vi "VI Tree.vi"   [LabVIEW 2020, in "Keysight DAQ970.lvlib"]
doc: "The VI Tree displays all the user-callable VIs of the instrument driver in an organized table."
uses:
  Keysight DAQ970.lvlib
panel:
  # "DAQ970"
  # "1.0.1"
  # "SEE DIAGRAM\nFOR VI Tree"
  # "© Keysight Technologies 2020 - 2021"
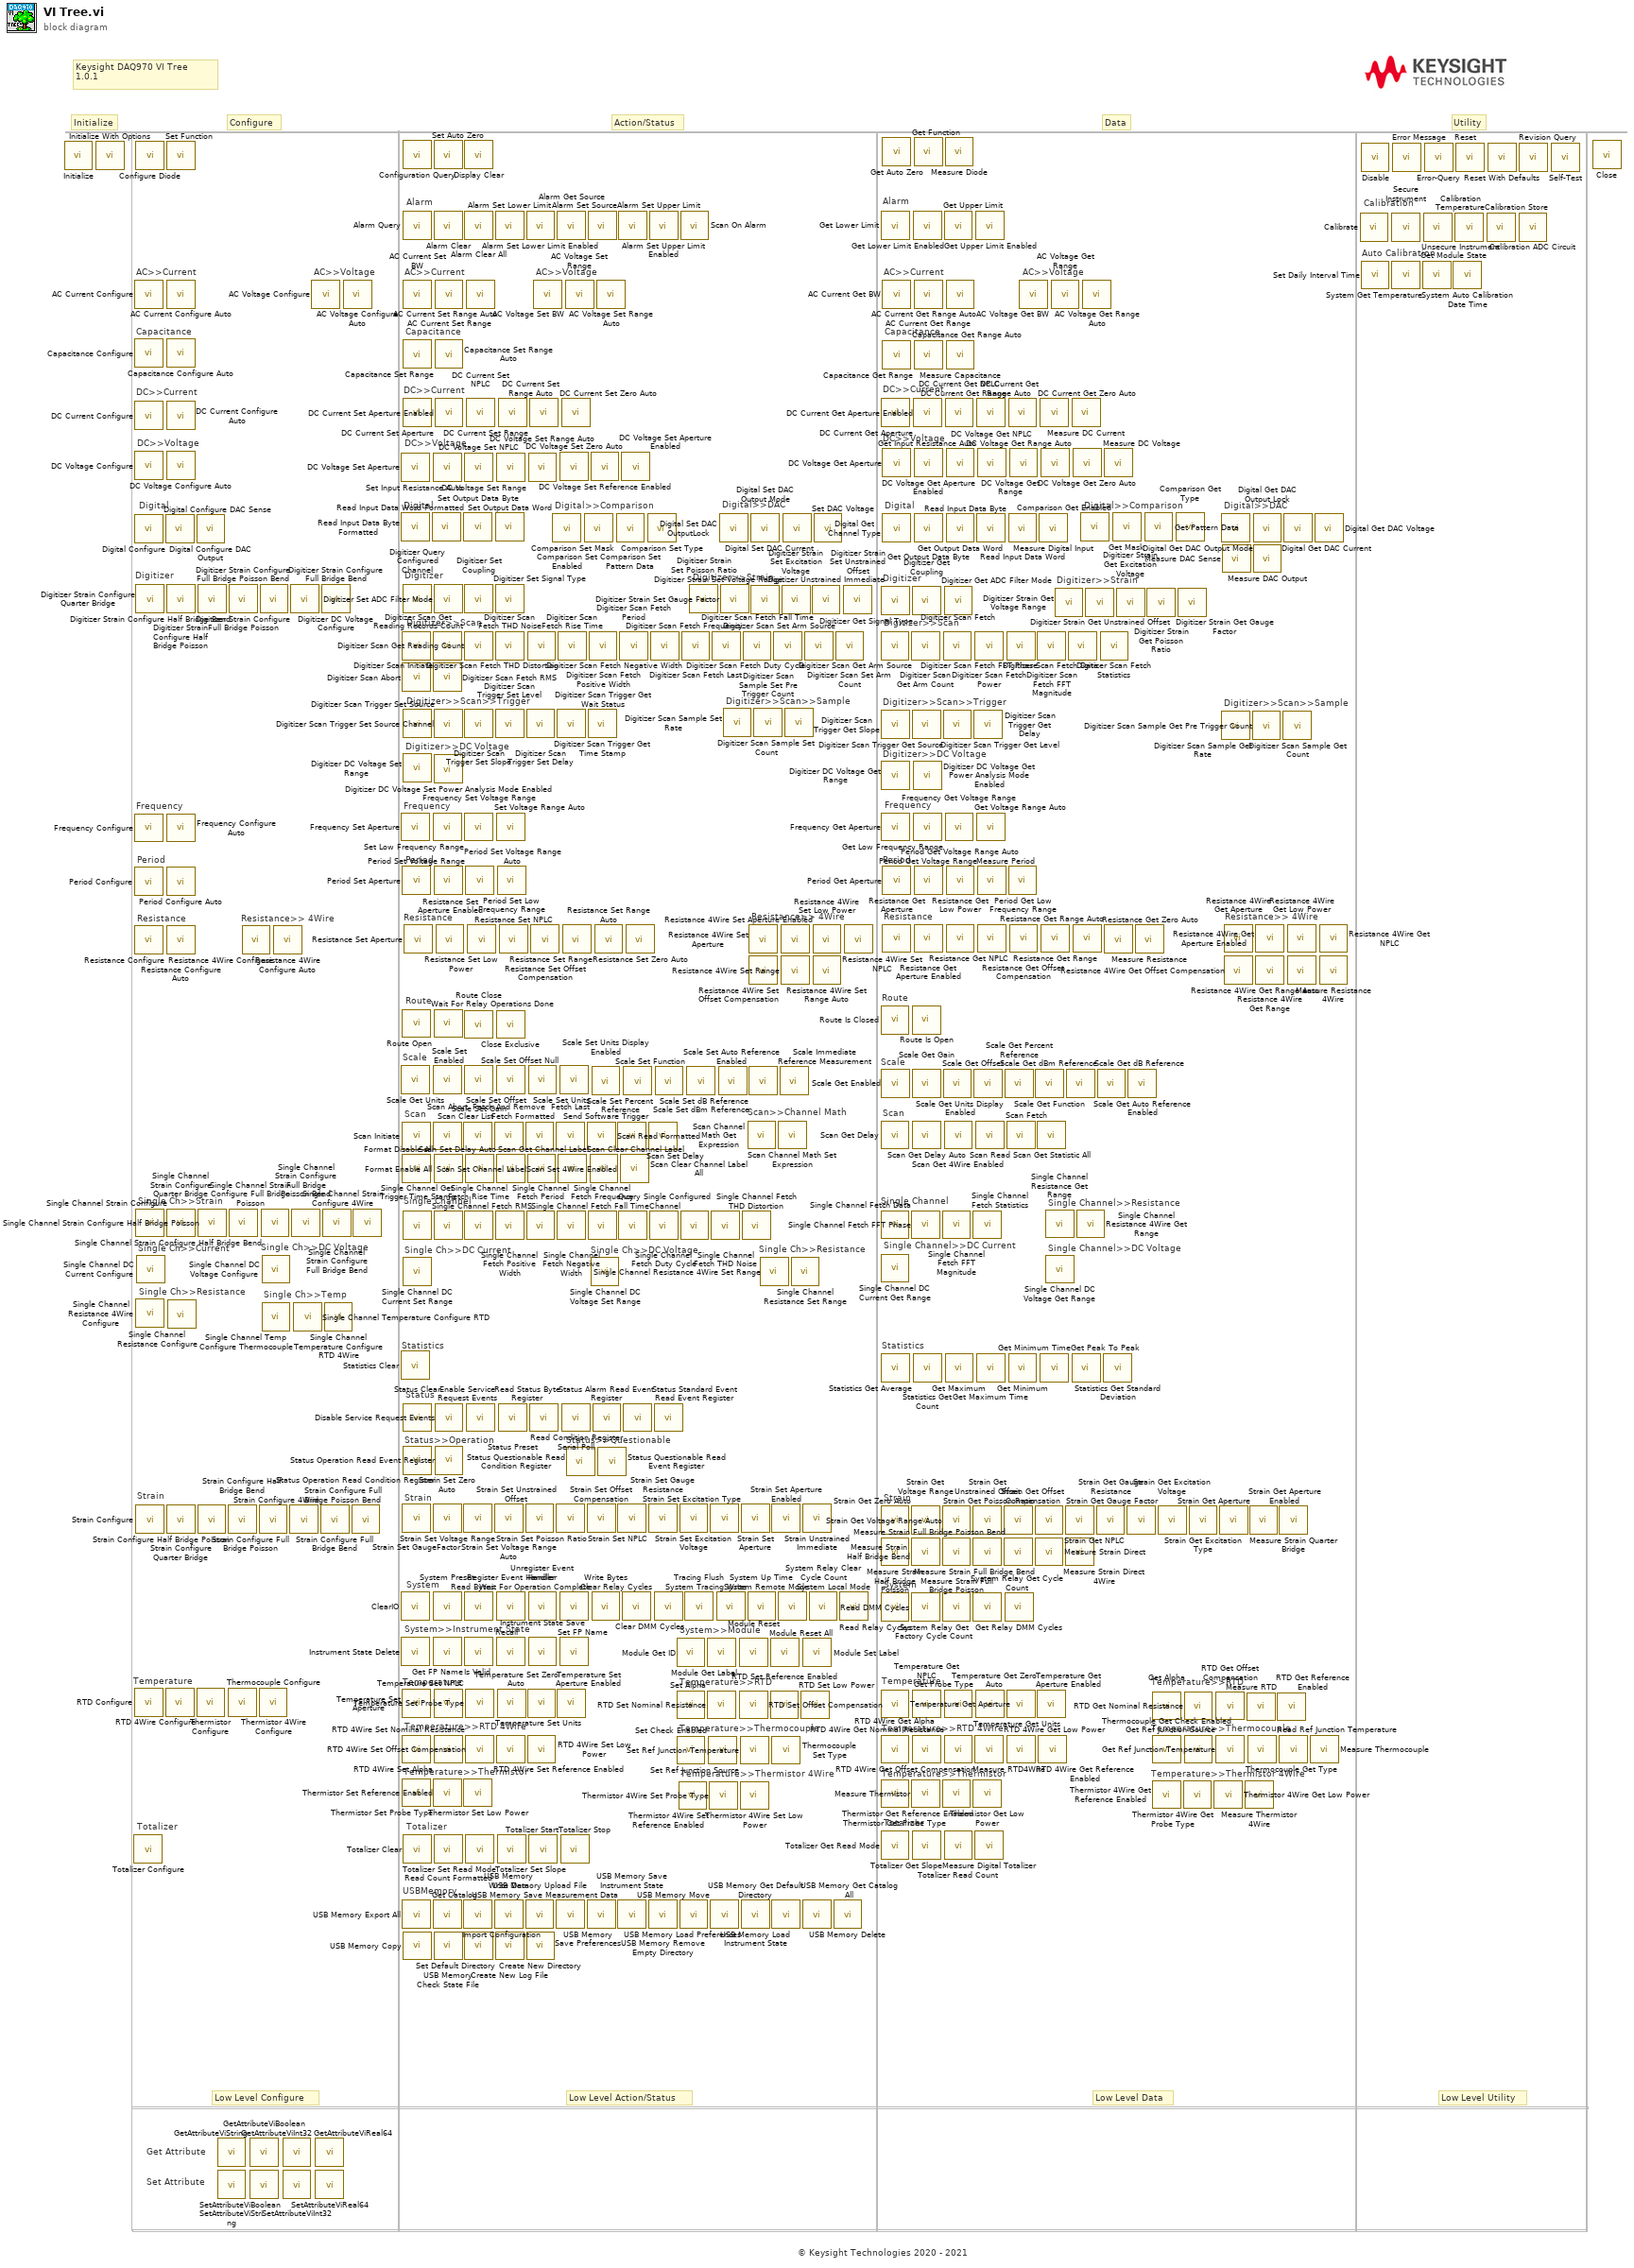
[diagram p0: block diagram]
diagram:
  # "Statistics"
  # "USBMemory"
  # "Totalizer"
  # "Totalizer"
  # "Temperature>>Thermistor"
  # "Temperature>>Thermistor 4Wire"
  # "Temperature>>Thermocouple"
  # "Temperature>>Thermistor 4Wire"
  # "Temperature>>Thermistor"
  # "Temperature>>Thermocouple"
  # "Temperature>>RTD 4Wire"
  # "Temperature>>RTD 4Wire"
  # "Temperature>>RTD"
  # "Temperature>>RTD"
  # "Temperature"
  # "Temperature"
  # "System>>Module"
  # "System>>Instrument State"
  # "Auto Calibration"
  # "System"
  # "System"
  # "Strain"
  # "Strain"
  # "Strain"
  # "Status>>Questionable"
  # "Status"
  # "Single Ch>>Temp"
  # "Single Ch>>Resistance"
  # "Single Ch>>DC Voltage"
  # "Single Ch>>Current"
  # "Single Ch>>Resistance"
  # "Single Channel>>DC Voltage"
  # "Single Channel>>Resistance"
  # "Single Ch>>DC Voltage"
  # "Single Channel>>DC Current"
  # "Single Ch>>DC Current"
  # "Single Ch>>Strain"
  # "Single Channel"
  # "Single Channel"
  # "Scan>>Channel Math"
  # "Scan"
  # "Scale"
  # "Scale"
  # "Route"
  # "Resistance>> 4Wire"
  # "Resistance>> 4Wire"
  # "Resistance>> 4Wire"
  # "Resistance"
  # "Resistance"
  # "Period"
  # "Period"
  # "Frequency"
  # "Frequency"
  # "Digitizer"
  # "Digitizer>>DC Voltage"
  # "Digitizer>>DC Voltage"
  # "Digitizer>>Scan>>Sample"
  # "Digitizer>>Scan>>Trigger"
  # "Digitizer>>Scan>>Sample"
  # "Digitizer>>Scan>>Trigger"
  # "Digitizer>>Scan"
  # "Digitizer>>Scan"
  # "Digitizer>>Strain"
  # "Digitizer"
  # "Digitizer>>Strain"
  # "Digitizer"
  # "Digital>>Comparison"
  # "Digital>>DAC"
  # "Digital>>DAC"
  # "Digital"
  # "Digital>>Comparison"
  # "Digital"
  # "DC>>Voltage"
  # "DC>>Voltage"
  # "DC>>Voltage"
  # "DC>>Current"
  # "DC>>Current"
  # "DC>>Current"
  # "Capacitance"
  # "Capacitance"
  # "AC>>Voltage"
  # "AC>>Voltage"
  # "AC>>Current"
  # "AC>>Current"
  # "Alarm"
  # "Set Attribute"
  # "Get Attribute"
  # "Low Level Utility"
  # "Low Level Configure"
  # "Low Level Action/Status"
  # "Low Level Data"
  # "© Keysight Technologies 2020 - 2021"
  # "Action/Status"
  # "Keysight DAQ970 VI Tree\n1.0.1"
  # "Utility"
  # "Data"
  # "Configure"
  # "Initialize"
  # "Status>>Operation"
  # "Statistics"
  # "Scan"
  # "Route"
  # "Temperature"
  # "Resistance"
  # "Period"
  # "Frequency"
  # "Totalizer"
  # "Digital"
  # "Capacitance"
  # "AC>>Voltage"
  # "AC>>Current"
  # "Calibration"
  # "Alarm"
  n1 = call "Initialize.vi"() -> ()  [unwired: 10 in, 2 out]
  n2 = call "Initialize With Options.vi"() -> ()  [unwired: 10 in, 2 out]
  n3 = call "Totalizer Configure.vi"() -> ()  [unwired: 10 in, 2 out]
  n4 = call "AC Current Configure.vi"() -> ()  [unwired: 10 in, 2 out]
  n5 = call "Capacitance Configure.vi"() -> ()  [unwired: 10 in, 2 out]
  n6 = call "DC Current Configure.vi"() -> ()  [unwired: 10 in, 2 out]
  n7 = call "DC Voltage Configure.vi"() -> ()  [unwired: 10 in, 2 out]
  n8 = call "Digital Configure.vi"() -> ()  [unwired: 10 in, 2 out]
  n9 = call "Frequency Configure.vi"() -> ()  [unwired: 10 in, 2 out]
  n10 = call "Period Configure.vi"() -> ()  [unwired: 10 in, 2 out]
  n11 = call "Resistance Configure.vi"() -> ()  [unwired: 10 in, 2 out]
  n12 = call "RTD Configure.vi"() -> ()  [unwired: 10 in, 2 out]
  n13 = call "Configure Diode.vi"() -> ()  [unwired: 10 in, 2 out]
  n14 = call "Digitizer Strain Configure Quarter Bridge.vi"() -> ()  [unwired: 14 in, 2 out]
  n15 = call "Single Channel Strain Configure.vi"() -> ()  [unwired: 10 in, 2 out]
  n16 = call "Single Channel Resistance 4Wire Configure.vi"() -> ()  [unwired: 10 in, 2 out]
  n17 = call "Strain Configure.vi"() -> ()  [unwired: 10 in, 2 out]
  n18 = call "Single Channel DC Current Configure.vi"() -> ()  [unwired: 10 in, 2 out]
  n19 = call "Digital Configure DAC Sense.vi"() -> ()  [unwired: 10 in, 2 out]
  n20 = call "RTD 4Wire Configure.vi"() -> ()  [unwired: 10 in, 2 out]
  n21 = call "Set Function.vi"() -> ()  [unwired: 10 in, 2 out]
  n22 = call "AC Current Configure Auto.vi"() -> ()  [unwired: 10 in, 2 out]
  n23 = call "Capacitance Configure Auto.vi"() -> ()  [unwired: 10 in, 2 out]
  n24 = call "DC Current Configure Auto.vi"() -> ()  [unwired: 10 in, 2 out]
  n25 = call "DC Voltage Configure Auto.vi"() -> ()  [unwired: 10 in, 2 out]
  n26 = call "Digitizer Strain Configure Half Bridge Poisson.vi"() -> ()  [unwired: 14 in, 2 out]
  n27 = call "Frequency Configure Auto.vi"() -> ()  [unwired: 10 in, 2 out]
  n28 = call "Period Configure Auto.vi"() -> ()  [unwired: 10 in, 2 out]
  n29 = call "Resistance Configure Auto.vi"() -> ()  [unwired: 10 in, 2 out]
  n30 = call "Single Channel Strain Configure Quarter Bridge.vi"() -> ()  [unwired: 10 in, 2 out]
  n31 = call "Strain Configure Quarter Bridge.vi"() -> ()  [unwired: 10 in, 2 out]
  n32 = call "Single Channel Resistance Configure.vi"() -> ()  [unwired: 10 in, 2 out]
  n33 = call "Digital Configure DAC Output.vi"() -> ()  [unwired: 10 in, 2 out]
  n34 = call "Thermistor Configure.vi"() -> ()  [unwired: 10 in, 2 out]
  n35 = call "Strain Configure Half Bridge Poisson.vi"() -> ()  [unwired: 10 in, 2 out]
  n36 = call "Digitizer Strain Configure Half Bridge Bend.vi"() -> ()  [unwired: 14 in, 2 out]
  n37 = call "Single Channel Strain Configure Half Bridge Poisson.vi"() -> ()  [unwired: 14 in, 2 out]
  n38 = call "GetAttributeViString.vi"() -> ()  [unwired: 9 in, 3 out]
  n39 = call "SetAttributeViString.vi"() -> ()  [unwired: 10 in, 2 out]
  n40 = call "Strain Configure Half Bridge Bend.vi"() -> ()  [unwired: 10 in, 2 out]
  n41 = call "Thermocouple Configure.vi"() -> ()  [unwired: 10 in, 2 out]
  n42 = call "Digitizer Strain Configure Full Bridge Poisson.vi"() -> ()  [unwired: 14 in, 2 out]
  n43 = call "Single Channel Strain Configure Half Bridge Bend.vi"() -> ()  [unwired: 10 in, 2 out]
  n44 = call "Resistance 4Wire Configure.vi"() -> ()  [unwired: 10 in, 2 out]
  n45 = call "GetAttributeViBoolean.vi"() -> ()  [unwired: 9 in, 3 out]
  n46 = call "SetAttributeViBoolean.vi"() -> ()  [unwired: 10 in, 2 out]
  n47 = call "Strain Configure Full Bridge Poisson.vi"() -> ()  [unwired: 14 in, 2 out]
  n48 = call "Thermistor 4Wire Configure.vi"() -> ()  [unwired: 10 in, 2 out]
  n49 = call "Digitizer Strain Configure Full Bridge Poisson Bend.vi"() -> ()  [unwired: 14 in, 2 out]
  n50 = call "Single Channel Strain Configure Full Bridge Poisson.vi"() -> ()  [unwired: 14 in, 2 out]
  n51 = call "Single Channel DC Voltage Configure.vi"() -> ()  [unwired: 10 in, 2 out]
  n52 = call "Single Channel Temp Configure Thermocouple.vi"() -> ()  [unwired: 10 in, 2 out]
  n53 = call "Resistance 4Wire Configure Auto.vi"() -> ()  [unwired: 10 in, 2 out]
  n54 = call "GetAttributeViInt32.vi"() -> ()  [unwired: 9 in, 3 out]
  n55 = call "SetAttributeViInt32.vi"() -> ()  [unwired: 10 in, 2 out]
  n56 = call "Strain Configure 4Wire.vi"() -> ()  [unwired: 10 in, 2 out]
  n57 = call "Digitizer Strain Configure Full Bridge Bend.vi"() -> ()  [unwired: 14 in, 2 out]
  n58 = call "Single Channel Strain Configure Full Bridge Poisson Bend.vi"() -> ()  [unwired: 14 in, 2 out]
  n59 = call "Single Channel Temperature Configure RTD.vi"() -> ()  [unwired: 10 in, 2 out]
  n60 = call "AC Voltage Configure.vi"() -> ()  [unwired: 10 in, 2 out]
  n61 = call "GetAttributeViReal64.vi"() -> ()  [unwired: 9 in, 3 out]
  n62 = call "SetAttributeViReal64.vi"() -> ()  [unwired: 10 in, 2 out]
  n63 = call "Strain Configure Full Bridge Bend.vi"() -> ()  [unwired: 10 in, 2 out]
  n64 = call "Digitizer DC Voltage Configure.vi"() -> ()  [unwired: 14 in, 2 out]
  n65 = call "Single Channel Strain Configure Full Bridge Bend.vi"() -> ()  [unwired: 10 in, 2 out]
  n66 = call "Single Channel Temperature Configure RTD 4Wire.vi"() -> ()  [unwired: 10 in, 2 out]
  n67 = call "AC Voltage Configure Auto.vi"() -> ()  [unwired: 10 in, 2 out]
  n68 = call "Strain Configure Full Bridge Poisson Bend.vi"() -> ()  [unwired: 10 in, 2 out]
  n69 = call "Single Channel Strain Configure 4Wire.vi"() -> ()  [unwired: 10 in, 2 out]
  n70 = call "DC Voltage Set Aperture.vi"() -> ()  [unwired: 10 in, 2 out]
  n71 = call "Read Input Data Byte Formatted.vi"() -> ()  [unwired: 9 in, 3 out]
  n72 = call "Frequency Set Aperture.vi"() -> ()  [unwired: 10 in, 2 out]
  n73 = call "Scale Get Units.vi"() -> ()  [unwired: 9 in, 3 out]
  n74 = call "Statistics Clear.vi"() -> ()  [unwired: 10 in, 2 out]
  n75 = call "ClearIO.vi"() -> ()  [unwired: 10 in, 2 out]
  n76 = call "Instrument State Delete.vi"() -> ()  [unwired: 10 in, 2 out]
  n77 = call "Digitizer Scan Initiate.vi"() -> ()  [unwired: 10 in, 2 out]
  n78 = call "Digitizer Scan Abort.vi"() -> ()  [unwired: 10 in, 2 out]
  n79 = call "Period Set Aperture.vi"() -> ()  [unwired: 10 in, 2 out]
  n80 = call "Route Open.vi"() -> ()  [unwired: 10 in, 2 out]
  n81 = call "Scan Initiate.vi"() -> ()  [unwired: 10 in, 2 out]
  n82 = call "Format Disable All.vi"() -> ()  [unwired: 10 in, 2 out]
  n83 = call "Strain Set GaugeFactor.vi"() -> ()  [unwired: 10 in, 2 out]
  n84 = call "Temperature Set Aperture.vi"() -> ()  [unwired: 10 in, 2 out]
  n85 = call "RTD 4Wire Set Alpha.vi"() -> ()  [unwired: 10 in, 2 out]
  n86 = call "Thermistor Set Probe Type.vi"() -> ()  [unwired: 10 in, 2 out]
  n87 = call "USB Memory Export All.vi"() -> ()  [unwired: 10 in, 2 out]
  n88 = call "Configuration Query.vi"() -> ()  [unwired: 9 in, 3 out]
  n89 = call "Alarm Query.vi"() -> ()  [unwired: 9 in, 3 out]
  n90 = call "AC Current Set BW.vi"() -> ()  [unwired: 10 in, 2 out]
  n91 = call "Capacitance Set Range.vi"() -> ()  [unwired: 10 in, 2 out]
  n92 = call "DC Current Set Aperture.vi"() -> ()  [unwired: 10 in, 2 out]
  n93 = call "Digitizer Query Configured Channel.vi"() -> ()  [unwired: 9 in, 3 out]
  n94 = call "Digitizer Scan Trigger Set Source.vi"() -> ()  [unwired: 10 in, 2 out]
  n95 = call "Digitizer DC Voltage Set Range.vi"() -> ()  [unwired: 10 in, 2 out]
  n96 = call "Single Channel Get Trigger Time Stamp.vi"() -> ()  [unwired: 9 in, 3 out]
  n97 = call "Single Channel DC Current Set Range.vi"() -> ()  [unwired: 10 in, 2 out]
  n98 = call "Status Clear.vi"() -> ()  [unwired: 10 in, 2 out]
  n99 = call "Status Operation Read Condition Register.vi"() -> ()  [unwired: 9 in, 3 out]
  n100 = call "Totalizer Clear.vi"() -> ()  [unwired: 10 in, 2 out]
  n101 = call "USB Memory Copy.vi"() -> ()  [unwired: 10 in, 2 out]
  n102 = call "Resistance Set Aperture.vi"() -> ()  [unwired: 10 in, 2 out]
  n103 = call "Read Input Data Word Formatted.vi"() -> ()  [unwired: 9 in, 3 out]
  n104 = call "Set Input Resistance Auto.vi"() -> ()  [unwired: 10 in, 2 out]
  n105 = call "Digitizer Scan Get Reading Records Count.vi"() -> ()  [unwired: 9 in, 3 out]
  n106 = call "Digitizer Scan Fetch RMS.vi"() -> ()  [unwired: 9 in, 3 out]
  n107 = call "Set Low Frequency Range.vi"() -> ()  [unwired: 10 in, 2 out]
  n108 = call "Scale Set Enabled.vi"() -> ()  [unwired: 10 in, 2 out]
  n109 = call "Scan Abort.vi"() -> ()  [unwired: 10 in, 2 out]
  n110 = call "Strain Set Zero Auto.vi"() -> ()  [unwired: 10 in, 2 out]
  n111 = call "System Preset.vi"() -> ()  [unwired: 10 in, 2 out]
  n112 = call "Get FP Name.vi"() -> ()  [unwired: 9 in, 3 out]
  n113 = call "Thermistor Set Reference Enabled.vi"() -> ()  [unwired: 10 in, 2 out]
  n114 = call "Get Catalog.vi"() -> ()  [unwired: 9 in, 3 out]
  n115 = call "Set Auto Zero.vi"() -> ()  [unwired: 10 in, 2 out]
  n116 = call "Alarm Clear.vi"() -> ()  [unwired: 10 in, 2 out]
  n117 = call "Digitizer Set ADC Filter Mode.vi"() -> ()  [unwired: 10 in, 2 out]
  n118 = call "Digitizer Scan Trigger Set Source Channel.vi"() -> ()  [unwired: 10 in, 2 out]
  n119 = call "Digitizer DC Voltage Set Power Analysis Mode Enabled.vi"() -> ()  [unwired: 10 in, 2 out]
  n120 = call "Period Set Voltage Range.vi"() -> ()  [unwired: 10 in, 2 out]
  n121 = call "Wait For Relay Operations Done.vi"() -> ()  [unwired: 10 in, 2 out]
  n122 = call "Format Enable All.vi"() -> ()  [unwired: 10 in, 2 out]
  n123 = call "Single Channel Fetch RMS.vi"() -> ()  [unwired: 9 in, 3 out]
  n124 = call "Temperature Set NPLC.vi"() -> ()  [unwired: 10 in, 2 out]
  n125 = call "RTD 4Wire Set Nominal Resistance.vi"() -> ()  [unwired: 10 in, 2 out]
  n126 = call "Read Count Formatted.vi"() -> ()  [unwired: 9 in, 3 out]
  n127 = call "USB Memory Check State File.vi"() -> ()  [unwired: 9 in, 3 out]
  n128 = call "AC Current Set Range.vi"() -> ()  [unwired: 10 in, 2 out]
  n129 = call "Capacitance Set Range Auto.vi"() -> ()  [unwired: 10 in, 2 out]
  n130 = call "DC Current Set Aperture Enabled.vi"() -> ()  [unwired: 10 in, 2 out]
  n131 = call "Disable Service Request Events.vi"() -> ()  [unwired: 10 in, 2 out]
  n132 = call "Status Operation Read Event Register.vi"() -> ()  [unwired: 9 in, 3 out]
  n133 = call "Resistance Set Aperture Enabled.vi"() -> ()  [unwired: 10 in, 2 out]
  n134 = call "Set Output Data Byte.vi"() -> ()  [unwired: 10 in, 2 out]
  n135 = call "Scan Clear List.vi"() -> ()  [unwired: 10 in, 2 out]
  n136 = call "Strain Set Voltage Range.vi"() -> ()  [unwired: 10 in, 2 out]
  n137 = call "Thermistor Set Low Power.vi"() -> ()  [unwired: 10 in, 2 out]
  n138 = call "Import Configuration.vi"() -> ()  [unwired: 10 in, 2 out]
  n139 = call "Display Clear.vi"() -> ()  [unwired: 10 in, 2 out]
  n140 = call "Alarm Clear All.vi"() -> ()  [unwired: 10 in, 2 out]
  n141 = call "DC Voltage Set NPLC.vi"() -> ()  [unwired: 10 in, 2 out]
  n142 = call "Digitizer Set Coupling.vi"() -> ()  [unwired: 10 in, 2 out]
  n143 = call "Digitizer Scan Get Reading Count.vi"() -> ()  [unwired: 9 in, 3 out]
  n144 = call "Digitizer Scan Trigger Set Slope.vi"() -> ()  [unwired: 10 in, 2 out]
  n145 = call "Frequency Set Voltage Range.vi"() -> ()  [unwired: 10 in, 2 out]
  n146 = call "Route Close.vi"() -> ()  [unwired: 10 in, 2 out]
  n147 = call "Scale Set Gain.vi"() -> ()  [unwired: 10 in, 2 out]
  n148 = call "Single Channel Fetch Rise Time.vi"() -> ()  [unwired: 9 in, 3 out]
  n149 = call "Read Bytes.vi"() -> ()  [unwired: 8 in, 4 out]
  n150 = call "Is Valid.vi"() -> ()  [unwired: 9 in, 3 out]
  n151 = call "Set Default Directory.vi"() -> ()  [unwired: 10 in, 2 out]
  n152 = call "Period Set Voltage Range Auto.vi"() -> ()  [unwired: 10 in, 2 out]
  n153 = call "Scan Set Delay Auto.vi"() -> ()  [unwired: 10 in, 2 out]
  n154 = call "Temperature Set Probe Type.vi"() -> ()  [unwired: 10 in, 2 out]
  n155 = call "RTD 4Wire Set Offset Compensation.vi"() -> ()  [unwired: 10 in, 2 out]
  n156 = call "Totalizer Set Read Mode.vi"() -> ()  [unwired: 10 in, 2 out]
  n157 = call "AC Current Set Range Auto.vi"() -> ()  [unwired: 10 in, 2 out]
  n158 = call "DC Current Set NPLC.vi"() -> ()  [unwired: 10 in, 2 out]
  n159 = call "Enable Service Request Events.vi"() -> ()  [unwired: 10 in, 2 out]
  n160 = call "Resistance Set Low Power.vi"() -> ()  [unwired: 10 in, 2 out]
  n161 = call "Fetch And Remove.vi"() -> ()  [unwired: 9 in, 3 out]
  n162 = call "Strain Set Voltage Range Auto.vi"() -> ()  [unwired: 10 in, 2 out]
  n163 = call "USB Memory Write Data.vi"() -> ()  [unwired: 10 in, 2 out]
  n164 = call "Alarm Set Lower Limit.vi"() -> ()  [unwired: 10 in, 2 out]
  n165 = call "Set Output Data Word.vi"() -> ()  [unwired: 10 in, 2 out]
  n166 = call "Digitizer Set Signal Type.vi"() -> ()  [unwired: 10 in, 2 out]
  n167 = call "Digitizer Scan Fetch THD Noise.vi"() -> ()  [unwired: 9 in, 3 out]
  n168 = call "Digitizer Scan Trigger Set Level.vi"() -> ()  [unwired: 10 in, 2 out]
  n169 = call "Single Channel Fetch Positive Width.vi"() -> ()  [unwired: 9 in, 3 out]
  n170 = call "Create New Log File.vi"() -> ()  [unwired: 10 in, 2 out]
  n171 = call "DC Voltage Set Range.vi"() -> ()  [unwired: 10 in, 2 out]
  n172 = call "Set Voltage Range Auto.vi"() -> ()  [unwired: 10 in, 2 out]
  n173 = call "Close Exclusive.vi"() -> ()  [unwired: 10 in, 2 out]
  n174 = call "Scale Set Offset.vi"() -> ()  [unwired: 10 in, 2 out]
  n175 = call "Scan Set 4Wire Enabled.vi"() -> ()  [unwired: 10 in, 2 out]
  n176 = call "Register Event Handler.vi"() -> ()  [unwired: 10 in, 2 out]
  n177 = call "Recall.vi"() -> ()  [unwired: 10 in, 2 out]
  n178 = call "RTD 4Wire Set Reference Enabled.vi"() -> ()  [unwired: 10 in, 2 out]
  n179 = call "Period Set Low Frequency Range.vi"() -> ()  [unwired: 10 in, 2 out]
  n180 = call "Temperature Set Units.vi"() -> ()  [unwired: 10 in, 2 out]
  n181 = call "Totalizer Set Slope.vi"() -> ()  [unwired: 10 in, 2 out]
  n182 = call "DC Current Set Range.vi"() -> ()  [unwired: 10 in, 2 out]
  n183 = call "Status Preset.vi"() -> ()  [unwired: 10 in, 2 out]
  n184 = call "Resistance Set NPLC.vi"() -> ()  [unwired: 10 in, 2 out]
  n185 = call "Fetch Formatted.vi"() -> ()  [unwired: 9 in, 3 out]
  n186 = call "Strain Set Unstrained Offset.vi"() -> ()  [unwired: 10 in, 2 out]
  n187 = call "USB Memory Upload File.vi"() -> ()  [unwired: 8 in, 4 out]
  n188 = call "Alarm Set Lower Limit Enabled.vi"() -> ()  [unwired: 10 in, 2 out]
  n189 = call "Digitizer Scan Trigger Set Delay.vi"() -> ()  [unwired: 10 in, 2 out]
  n190 = call "Single Channel Fetch Period.vi"() -> ()  [unwired: 9 in, 3 out]
  n191 = call "Create New Directory.vi"() -> ()  [unwired: 10 in, 2 out]
  n192 = call "Digitizer Scan Fetch THD Distortion.vi"() -> ()  [unwired: 9 in, 3 out]
  n193 = call "Scan Set Channel Label.vi"() -> ()  [unwired: 10 in, 2 out]
  n194 = call "Temperature Set Zero Auto.vi"() -> ()  [unwired: 10 in, 2 out]
  n195 = call "RTD 4Wire Set Low Power.vi"() -> ()  [unwired: 10 in, 2 out]
  n196 = call "DC Voltage Set Range Auto.vi"() -> ()  [unwired: 10 in, 2 out]
  n197 = call "Scale Set Offset Null.vi"() -> ()  [unwired: 10 in, 2 out]
  n198 = call "Unregister Event Handler.vi"() -> ()  [unwired: 10 in, 2 out]
  n199 = call "Instrument State Save.vi"() -> ()  [unwired: 10 in, 2 out]
  n200 = call "Totalizer Start.vi"() -> ()  [unwired: 10 in, 2 out]
  n201 = call "DC Current Set Range Auto.vi"() -> ()  [unwired: 10 in, 2 out]
  n202 = call "Read Status Byte Register.vi"() -> ()  [unwired: 9 in, 3 out]
  n203 = call "Resistance Set Offset Compensation.vi"() -> ()  [unwired: 10 in, 2 out]
  n204 = call "AC Voltage Set BW.vi"() -> ()  [unwired: 10 in, 2 out]
  n205 = call "Comparison Set Enabled.vi"() -> ()  [unwired: 10 in, 2 out]
  n206 = call "Fetch Last.vi"() -> ()  [unwired: 9 in, 3 out]
  n207 = call "Strain Set Poisson Ratio.vi"() -> ()  [unwired: 10 in, 2 out]
  n208 = call "USB Memory Save Preferences.vi"() -> ()  [unwired: 10 in, 2 out]
  n209 = call "Alarm Get Source.vi"() -> ()  [unwired: 9 in, 3 out]
  n210 = call "Digitizer Scan Trigger Get Wait Status.vi"() -> ()  [unwired: 9 in, 3 out]
  n211 = call "Single Channel Fetch Negative Width.vi"() -> ()  [unwired: 9 in, 3 out]
  n212 = call "Temperature Set Aperture Enabled.vi"() -> ()  [unwired: 10 in, 2 out]
  n213 = call "Digitizer Scan Fetch Rise Time.vi"() -> ()  [unwired: 9 in, 3 out]
  n214 = call "Scan Get Channel Label.vi"() -> ()  [unwired: 9 in, 3 out]
  n215 = call "DC Voltage Set Zero Auto.vi"() -> ()  [unwired: 10 in, 2 out]
  n216 = call "Scale Set Units.vi"() -> ()  [unwired: 10 in, 2 out]
  n217 = call "Wait For Operation Complete.vi"() -> ()  [unwired: 10 in, 2 out]
  n218 = call "Set FP Name.vi"() -> ()  [unwired: 10 in, 2 out]
  n219 = call "Totalizer Stop.vi"() -> ()  [unwired: 10 in, 2 out]
  n220 = call "DC Current Set Zero Auto.vi"() -> ()  [unwired: 10 in, 2 out]
  n221 = call "Serial Poll.vi"() -> ()  [unwired: 9 in, 3 out]
  n222 = call "Resistance Set Range.vi"() -> ()  [unwired: 10 in, 2 out]
  n223 = call "AC Voltage Set Range.vi"() -> ()  [unwired: 10 in, 2 out]
  n224 = call "Status Questionable Read Condition Register.vi"() -> ()  [unwired: 9 in, 3 out]
  n225 = call "Comparison Set Mask.vi"() -> ()  [unwired: 10 in, 2 out]
  n226 = call "Scan Read Formatted.vi"() -> ()  [unwired: 9 in, 3 out]
  n227 = call "Strain Set Offset Compensation.vi"() -> ()  [unwired: 10 in, 2 out]
  n228 = call "USB Memory Save Measurement Data.vi"() -> ()  [unwired: 10 in, 2 out]
  n229 = call "Alarm Set Source.vi"() -> ()  [unwired: 10 in, 2 out]
  n230 = call "Digitizer Scan Trigger Get Time Stamp.vi"() -> ()  [unwired: 9 in, 3 out]
  n231 = call "Single Channel Fetch Frequency.vi"() -> ()  [unwired: 9 in, 3 out]
  n232 = call "Digitizer Scan Fetch Positive Width.vi"() -> ()  [unwired: 9 in, 3 out]
  n233 = call "Scan Clear Channel Label.vi"() -> ()  [unwired: 10 in, 2 out]
  n234 = call "DC Voltage Set Reference Enabled.vi"() -> ()  [unwired: 10 in, 2 out]
  n235 = call "Single Channel DC Voltage Set Range.vi"() -> ()  [unwired: 10 in, 2 out]
  n236 = call "Scale Set Units Display Enabled.vi"() -> ()  [unwired: 10 in, 2 out]
  n237 = call "Write Bytes.vi"() -> ()  [unwired: 9 in, 3 out]
  n238 = call "Read Condition Register.vi"() -> ()  [unwired: 9 in, 3 out]
  n239 = call "Resistance Set Range Auto.vi"() -> ()  [unwired: 10 in, 2 out]
  n240 = call "AC Voltage Set Range Auto.vi"() -> ()  [unwired: 10 in, 2 out]
  n241 = call "Status Questionable Read Event Register.vi"() -> ()  [unwired: 9 in, 3 out]
  n242 = call "Comparison Set Pattern Data.vi"() -> ()  [unwired: 10 in, 2 out]
  n243 = call "Send Software Trigger.vi"() -> ()  [unwired: 10 in, 2 out]
  n244 = call "Strain Set NPLC.vi"() -> ()  [unwired: 10 in, 2 out]
  n245 = call "USB Memory Save Instrument State.vi"() -> ()  [unwired: 10 in, 2 out]
  n246 = call "Alarm Set Upper Limit.vi"() -> ()  [unwired: 10 in, 2 out]
  n247 = call "Single Channel Fetch Fall Time.vi"() -> ()  [unwired: 9 in, 3 out]
  n248 = call "Digitizer Scan Fetch Period.vi"() -> ()  [unwired: 9 in, 3 out]
  n249 = call "Scan Clear Channel Label All.vi"() -> ()  [unwired: 10 in, 2 out]
  n250 = call "DC Voltage Set Aperture Enabled.vi"() -> ()  [unwired: 10 in, 2 out]
  n251 = call "Clear Relay Cycles.vi"() -> ()  [unwired: 10 in, 2 out]
  n252 = call "Scale Set Percent Reference.vi"() -> ()  [unwired: 10 in, 2 out]
  n253 = call "Status Alarm Read Event Register.vi"() -> ()  [unwired: 9 in, 3 out]
  n254 = call "Resistance Set Zero Auto.vi"() -> ()  [unwired: 10 in, 2 out]
  n255 = call "Comparison Set Type.vi"() -> ()  [unwired: 10 in, 2 out]
  n256 = call "Scan Set Delay.vi"() -> ()  [unwired: 10 in, 2 out]
  n257 = call "Strain Set Gauge Resistance.vi"() -> ()  [unwired: 10 in, 2 out]
  n258 = call "USB Memory Remove Empty Directory.vi"() -> ()  [unwired: 10 in, 2 out]
  n259 = call "Alarm Set Upper Limit Enabled.vi"() -> ()  [unwired: 10 in, 2 out]
  n260 = call "Single Channel Fetch Duty Cycle.vi"() -> ()  [unwired: 9 in, 3 out]
  n261 = call "Digitizer Scan Fetch Negative Width.vi"() -> ()  [unwired: 9 in, 3 out]
  n262 = call "Status Standard Event Read Event Register.vi"() -> ()  [unwired: 9 in, 3 out]
  n263 = call "Clear DMM Cycles.vi"() -> ()  [unwired: 10 in, 2 out]
  n264 = call "Scale Set Function.vi"() -> ()  [unwired: 10 in, 2 out]
  n265 = call "Module Get ID.vi"() -> ()  [unwired: 9 in, 3 out]
  n266 = call "Set Alpha.vi"() -> ()  [unwired: 10 in, 2 out]
  n267 = call "Set Check Enabled.vi"() -> ()  [unwired: 10 in, 2 out]
  n268 = call "Thermistor 4Wire Set Reference Enabled.vi"() -> ()  [unwired: 10 in, 2 out]
  n269 = call "Strain Set Excitation Voltage.vi"() -> ()  [unwired: 10 in, 2 out]
  n270 = call "USB Memory Move.vi"() -> ()  [unwired: 10 in, 2 out]
  n271 = call "Scan On Alarm.vi"() -> ()  [unwired: 10 in, 2 out]
  n272 = call "Query Single Configured Channel.vi"() -> ()  [unwired: 9 in, 3 out]
  n273 = call "Digitizer Scan Fetch Last.vi"() -> ()  [unwired: 8 in, 4 out]
  n274 = call "Tracing Flush.vi"() -> ()  [unwired: 10 in, 2 out]
  n275 = call "Scale Set dBm Reference.vi"() -> ()  [unwired: 10 in, 2 out]
  n276 = call "Digitizer Strain Set Poisson Ratio.vi"() -> ()  [unwired: 10 in, 2 out]
  n277 = call "Module Get Label.vi"() -> ()  [unwired: 9 in, 3 out]
  n278 = call "RTD Set Nominal Resistance.vi"() -> ()  [unwired: 10 in, 2 out]
  n279 = call "Set Ref Junction Source.vi"() -> ()  [unwired: 10 in, 2 out]
  n280 = call "Thermistor 4Wire Set Probe Type.vi"() -> ()  [unwired: 10 in, 2 out]
  n281 = call "Strain Set Excitation Type.vi"() -> ()  [unwired: 10 in, 2 out]
  n282 = call "USB Memory Load Preferences.vi"() -> ()  [unwired: 10 in, 2 out]
  n283 = call "Single Channel Fetch THD Noise.vi"() -> ()  [unwired: 9 in, 3 out]
  n284 = call "Digitizer Scan Fetch Frequency.vi"() -> ()  [unwired: 9 in, 3 out]
  n285 = call "System Tracing Write.vi"() -> ()  [unwired: 10 in, 2 out]
  n286 = call "Scale Set dB Reference.vi"() -> ()  [unwired: 10 in, 2 out]
  n287 = call "Digital Set DAC OutputLock.vi"() -> ()  [unwired: 10 in, 2 out]
  n288 = call "Digitizer Strain Set Gauge Factor.vi"() -> ()  [unwired: 10 in, 2 out]
  n289 = call "Digitizer Scan Sample Set Rate.vi"() -> ()  [unwired: 10 in, 2 out]
  n290 = call "Module Reset.vi"() -> ()  [unwired: 10 in, 2 out]
  n291 = call "RTD Set Offset Compensation.vi"() -> ()  [unwired: 10 in, 2 out]
  n292 = call "Set Ref Junction Temperature.vi"() -> ()  [unwired: 10 in, 2 out]
  n293 = call "Thermistor 4Wire Set Low Power.vi"() -> ()  [unwired: 10 in, 2 out]
  n294 = call "Strain Set Aperture.vi"() -> ()  [unwired: 10 in, 2 out]
  n295 = call "USB Memory Load Instrument State.vi"() -> ()  [unwired: 10 in, 2 out]
  n296 = call "Single Channel Fetch THD Distortion.vi"() -> ()  [unwired: 9 in, 3 out]
  n297 = call "Digitizer Scan Fetch Fall Time.vi"() -> ()  [unwired: 9 in, 3 out]
  n298 = call "Scan Channel Math Get Expression.vi"() -> ()  [unwired: 9 in, 3 out]
  n299 = call "System Up Time.vi"() -> ()  [unwired: 9 in, 3 out]
  n300 = call "Resistance 4Wire Set Aperture.vi"() -> ()  [unwired: 10 in, 2 out]
  n301 = call "Resistance 4Wire Set Offset Compensation.vi"() -> ()  [unwired: 10 in, 2 out]
  n302 = call "Scale Set Auto Reference Enabled.vi"() -> ()  [unwired: 10 in, 2 out]
  n303 = call "Digital Set DAC Output Mode.vi"() -> ()  [unwired: 10 in, 2 out]
  n304 = call "Digitizer Strain Set Voltage Range.vi"() -> ()  [unwired: 10 in, 2 out]
  n305 = call "Digitizer Scan Sample Set Pre Trigger Count.vi"() -> ()  [unwired: 10 in, 2 out]
  n306 = call "Single Channel Resistance 4Wire Set Range.vi"() -> ()  [unwired: 10 in, 2 out]
  n307 = call "RTD Set Reference Enabled.vi"() -> ()  [unwired: 10 in, 2 out]
  n308 = call "Module Reset All.vi"() -> ()  [unwired: 10 in, 2 out]
  n309 = call "Strain Set Aperture Enabled.vi"() -> ()  [unwired: 10 in, 2 out]
  n310 = call "Thermocouple Set Type.vi"() -> ()  [unwired: 10 in, 2 out]
  n311 = call "USB Memory Get Default Directory.vi"() -> ()  [unwired: 9 in, 3 out]
  n312 = call "Digitizer Scan Fetch Duty Cycle.vi"() -> ()  [unwired: 9 in, 3 out]
  n313 = call "Scan Channel Math Set Expression.vi"() -> ()  [unwired: 10 in, 2 out]
  n314 = call "System Remote Mode.vi"() -> ()  [unwired: 10 in, 2 out]
  n315 = call "Scale Immediate Reference Measurement.vi"() -> ()  [unwired: 10 in, 2 out]
  n316 = call "Resistance 4Wire Set Aperture Enabled.vi"() -> ()  [unwired: 10 in, 2 out]
  n317 = call "Resistance 4Wire Set Range.vi"() -> ()  [unwired: 10 in, 2 out]
  n318 = call "Digitizer Strain Set Excitation Voltage.vi"() -> ()  [unwired: 10 in, 2 out]
  n319 = call "Digital Set DAC Current.vi"() -> ()  [unwired: 10 in, 2 out]
  n320 = call "Digitizer Scan Sample Set Count.vi"() -> ()  [unwired: 10 in, 2 out]
  n321 = call "Single Channel Resistance Set Range.vi"() -> ()  [unwired: 10 in, 2 out]
  n322 = call "RTD Set Low Power.vi"() -> ()  [unwired: 10 in, 2 out]
  n323 = call "Strain Unstrained Immediate.vi"() -> ()  [unwired: 10 in, 2 out]
  n324 = call "Module Set Label.vi"() -> ()  [unwired: 10 in, 2 out]
  n325 = call "USB Memory Get Catalog All.vi"() -> ()  [unwired: 7 in, 5 out]
  n326 = call "Digitizer Scan Set Arm Source.vi"() -> ()  [unwired: 10 in, 2 out]
  n327 = call "System Relay Clear Cycle Count.vi"() -> ()  [unwired: 10 in, 2 out]
  n328 = call "Digitizer Unstrained Immediate.vi"() -> ()  [unwired: 10 in, 2 out]
  n329 = call "Resistance 4Wire Set Low Power.vi"() -> ()  [unwired: 10 in, 2 out]
  n330 = call "Resistance 4Wire Set Range Auto.vi"() -> ()  [unwired: 10 in, 2 out]
  n331 = call "Set DAC Voltage.vi"() -> ()  [unwired: 10 in, 2 out]
  n332 = call "USB Memory Delete.vi"() -> ()  [unwired: 10 in, 2 out]
  n333 = call "Digitizer Scan Set Arm Count.vi"() -> ()  [unwired: 10 in, 2 out]
  n334 = call "System Local Mode.vi"() -> ()  [unwired: 10 in, 2 out]
  n335 = call "Digitizer Strain Set Unstrained Offset.vi"() -> ()  [unwired: 10 in, 2 out]
  n336 = call "Resistance 4Wire Set NPLC.vi"() -> ()  [unwired: 10 in, 2 out]
  n337 = call "Digitizer Scan Get Arm Source.vi"() -> ()  [unwired: 8 in, 4 out]
  n338 = call "Route Is Closed.vi"() -> ()  [unwired: 8 in, 4 out]
  n339 = call "Scan Get Delay.vi"() -> ()  [unwired: 8 in, 4 out]
  n340 = call "Single Channel Fetch Data.vi"() -> ()  [unwired: 8 in, 4 out]
  n341 = call "Single Channel DC Current Get Range.vi"() -> ()  [unwired: 8 in, 4 out]
  n342 = call "Strain Get Zero Auto.vi"() -> ()  [unwired: 8 in, 4 out]
  n343 = call "Measure Strain Half Bridge Poisson.vi"() -> ()  [unwired: 8 in, 4 out]
  n344 = call "Read Relay Cycles.vi"() -> ()  [unwired: 8 in, 4 out]
  n345 = call "Temperature Get Aperture.vi"() -> ()  [unwired: 8 in, 4 out]
  n346 = call "RTD 4Wire Get Alpha.vi"() -> ()  [unwired: 8 in, 4 out]
  n347 = call "Thermistor Get Probe Type.vi"() -> ()  [unwired: 8 in, 4 out]
  n348 = call "Totalizer Get Read Mode.vi"() -> ()  [unwired: 8 in, 4 out]
  n349 = call "Get Lower Limit.vi"() -> ()  [unwired: 8 in, 4 out]
  n350 = call "DC Current Get Aperture.vi"() -> ()  [unwired: 8 in, 4 out]
  n351 = call "Digitizer Get Signal Type.vi"() -> ()  [unwired: 8 in, 4 out]
  n352 = call "Digitizer Scan Trigger Get Slope.vi"() -> ()  [unwired: 8 in, 4 out]
  n353 = call "Digitizer DC Voltage Get Range.vi"() -> ()  [unwired: 8 in, 4 out]
  n354 = call "Frequency Get Aperture.vi"() -> ()  [unwired: 8 in, 4 out]
  n355 = call "Scale Get Enabled.vi"() -> ()  [unwired: 8 in, 4 out]
  n356 = call "Statistics Get Average.vi"() -> ()  [unwired: 8 in, 4 out]
  n357 = call "Get Auto Zero.vi"() -> ()  [unwired: 8 in, 4 out]
  n358 = call "AC Current Get BW.vi"() -> ()  [unwired: 8 in, 4 out]
  n359 = call "Capacitance Get Range.vi"() -> ()  [unwired: 8 in, 4 out]
  n360 = call "DC Voltage Get Aperture.vi"() -> ()  [unwired: 8 in, 4 out]
  n361 = call "Digital Get Channel Type.vi"() -> ()  [unwired: 8 in, 4 out]
  n362 = call "Period Get Aperture.vi"() -> ()  [unwired: 8 in, 4 out]
  n363 = call "Resistance Get Aperture.vi"() -> ()  [unwired: 8 in, 4 out]
  n364 = call "Digitizer Scan Get Arm Count.vi"() -> ()  [unwired: 8 in, 4 out]
  n365 = call "Single Channel Fetch FFT Phase.vi"() -> ()  [unwired: 8 in, 4 out]
  n366 = call "Strain Get Voltage Range.vi"() -> ()  [unwired: 8 in, 4 out]
  n367 = call "Measure Strain Half Bridge Bend.vi"() -> ()  [unwired: 8 in, 4 out]
  n368 = call "Read DMM Cycles.vi"() -> ()  [unwired: 8 in, 4 out]
  n369 = call "Measure Thermistor.vi"() -> ()  [unwired: 8 in, 4 out]
  n370 = call "Digitizer Get Coupling.vi"() -> ()  [unwired: 8 in, 4 out]
  n371 = call "Digitizer Scan Trigger Get Source.vi"() -> ()  [unwired: 8 in, 4 out]
  n372 = call "Route Is Open.vi"() -> ()  [unwired: 8 in, 4 out]
  n373 = call "Scale Get Gain.vi"() -> ()  [unwired: 8 in, 4 out]
  n374 = call "Scan Get Delay Auto.vi"() -> ()  [unwired: 8 in, 4 out]
  n375 = call "Temperature Get NPLC.vi"() -> ()  [unwired: 8 in, 4 out]
  n376 = call "RTD 4Wire Get Nominal Resistance.vi"() -> ()  [unwired: 8 in, 4 out]
  n377 = call "Totalizer Get Slope.vi"() -> ()  [unwired: 8 in, 4 out]
  n378 = call "Get Lower Limit Enabled.vi"() -> ()  [unwired: 8 in, 4 out]
  n379 = call "DC Current Get Aperture Enabled.vi"() -> ()  [unwired: 8 in, 4 out]
  n380 = call "Digitizer DC Voltage Get Power Analysis Mode Enabled.vi"() -> ()  [unwired: 8 in, 4 out]
  n381 = call "Get Low Frequency Range.vi"() -> ()  [unwired: 8 in, 4 out]
  n382 = call "Statistics Get Count.vi"() -> ()  [unwired: 8 in, 4 out]
  n383 = call "Get Function.vi"() -> ()  [unwired: 8 in, 4 out]
  n384 = call "AC Current Get Range.vi"() -> ()  [unwired: 8 in, 4 out]
  n385 = call "Capacitance Get Range Auto.vi"() -> ()  [unwired: 8 in, 4 out]
  n386 = call "DC Voltage Get Aperture Enabled.vi"() -> ()  [unwired: 8 in, 4 out]
  n387 = call "Get Output Data Byte.vi"() -> ()  [unwired: 8 in, 4 out]
  n388 = call "Period Get Voltage Range.vi"() -> ()  [unwired: 8 in, 4 out]
  n389 = call "Resistance Get Aperture Enabled.vi"() -> ()  [unwired: 8 in, 4 out]
  n390 = call "Single Channel Fetch FFT Magnitude.vi"() -> ()  [unwired: 8 in, 4 out]
  n391 = call "Strain Get Voltage Range Auto.vi"() -> ()  [unwired: 8 in, 4 out]
  n392 = call "Measure Strain Full Bridge Poisson.vi"() -> ()  [unwired: 8 in, 4 out]
  n393 = call "System Relay Get Factory Cycle Count.vi"() -> ()  [unwired: 8 in, 4 out]
  n394 = call "Thermistor Get Reference Enabled.vi"() -> ()  [unwired: 8 in, 4 out]
  n395 = call "Digitizer Scan Fetch.vi"() -> ()  [unwired: 8 in, 4 out]
  n396 = call "Digitizer Scan Trigger Get Level.vi"() -> ()  [unwired: 8 in, 4 out]
  n397 = call "Scale Get Offset.vi"() -> ()  [unwired: 8 in, 4 out]
  n398 = call "Get Upper Limit.vi"() -> ()  [unwired: 8 in, 4 out]
  n399 = call "Digitizer Get ADC Filter Mode.vi"() -> ()  [unwired: 8 in, 4 out]
  n400 = call "Scan Get 4Wire Enabled.vi"() -> ()  [unwired: 8 in, 4 out]
  n401 = call "Get Probe Type.vi"() -> ()  [unwired: 8 in, 4 out]
  n402 = call "RTD 4Wire Get Offset Compensation.vi"() -> ()  [unwired: 8 in, 4 out]
  n403 = call "Totalizer Read Count.vi"() -> ()  [unwired: 8 in, 4 out]
  n404 = call "Measure Diode.vi"() -> ()  [unwired: 8 in, 4 out]
  n405 = call "DC Current Get NPLC.vi"() -> ()  [unwired: 8 in, 4 out]
  n406 = call "Frequency Get Voltage Range.vi"() -> ()  [unwired: 8 in, 4 out]
  n407 = call "Get Maximum.vi"() -> ()  [unwired: 8 in, 4 out]
  n408 = call "AC Current Get Range Auto.vi"() -> ()  [unwired: 8 in, 4 out]
  n409 = call "Measure Capacitance.vi"() -> ()  [unwired: 8 in, 4 out]
  n410 = call "Get Input Resistance Auto.vi"() -> ()  [unwired: 8 in, 4 out]
  n411 = call "Get Output Data Word.vi"() -> ()  [unwired: 8 in, 4 out]
  n412 = call "Period Get Voltage Range Auto.vi"() -> ()  [unwired: 8 in, 4 out]
  n413 = call "Resistance Get Low Power.vi"() -> ()  [unwired: 8 in, 4 out]
  n414 = call "Single Channel Fetch Statistics.vi"() -> ()  [unwired: 8 in, 4 out]
  n415 = call "Strain Get Unstrained Offset.vi"() -> ()  [unwired: 8 in, 4 out]
  n416 = call "Measure Strain Full Bridge Poisson Bend.vi"() -> ()  [unwired: 8 in, 4 out]
  n417 = call "System Relay Get Cycle Count.vi"() -> ()  [unwired: 8 in, 4 out]
  n418 = call "Thermistor Get Low Power.vi"() -> ()  [unwired: 8 in, 4 out]
  n419 = call "Digitizer Scan Trigger Get Delay.vi"() -> ()  [unwired: 8 in, 4 out]
  n420 = call "Scale Get Units Display Enabled.vi"() -> ()  [unwired: 8 in, 4 out]
  n421 = call "Digitizer Scan Fetch Power.vi"() -> ()  [unwired: 12 in, 4 out]
  n422 = call "Measure RTD4Wire.vi"() -> ()  [unwired: 8 in, 4 out]
  n423 = call "Measure Digital Totalizer.vi"() -> ()  [unwired: 8 in, 4 out]
  n424 = call "Get Upper Limit Enabled.vi"() -> ()  [unwired: 8 in, 4 out]
  n425 = call "Scan Read.vi"() -> ()  [unwired: 8 in, 4 out]
  n426 = call "Temperature Get Units.vi"() -> ()  [unwired: 8 in, 4 out]
  n427 = call "DC Current Get Range.vi"() -> ()  [unwired: 8 in, 4 out]
  n428 = call "Read Input Data Byte.vi"() -> ()  [unwired: 8 in, 4 out]
  n429 = call "Get Voltage Range Auto.vi"() -> ()  [unwired: 8 in, 4 out]
  n430 = call "Get Maximum Time.vi"() -> ()  [unwired: 8 in, 4 out]
  n431 = call "DC Voltage Get NPLC.vi"() -> ()  [unwired: 8 in, 4 out]
  n432 = call "Measure Period.vi"() -> ()  [unwired: 8 in, 4 out]
  n433 = call "Resistance Get NPLC.vi"() -> ()  [unwired: 8 in, 4 out]
  n434 = call "Strain Get Poisson Ratio.vi"() -> ()  [unwired: 8 in, 4 out]
  n435 = call "Measure Strain Full Bridge Bend.vi"() -> ()  [unwired: 8 in, 4 out]
  n436 = call "Scale Get Percent Reference.vi"() -> ()  [unwired: 8 in, 4 out]
  n437 = call "Get Relay DMM Cycles.vi"() -> ()  [unwired: 8 in, 4 out]
  n438 = call "Digitizer Scan Fetch FFT Phase.vi"() -> ()  [unwired: 12 in, 4 out]
  n439 = call "Scan Fetch.vi"() -> ()  [unwired: 8 in, 4 out]
  n440 = call "Temperature Get Zero Auto.vi"() -> ()  [unwired: 8 in, 4 out]
  n441 = call "RTD 4Wire Get Low Power.vi"() -> ()  [unwired: 8 in, 4 out]
  n442 = call "DC Current Get Range Auto.vi"() -> ()  [unwired: 8 in, 4 out]
  n443 = call "Read Input Data Word.vi"() -> ()  [unwired: 8 in, 4 out]
  n444 = call "Period Get Low Frequency Range.vi"() -> ()  [unwired: 8 in, 4 out]
  n445 = call "Get Minimum.vi"() -> ()  [unwired: 8 in, 4 out]
  n446 = call "DC Voltage Get Range.vi"() -> ()  [unwired: 8 in, 4 out]
  n447 = call "Resistance Get Offset Compensation.vi"() -> ()  [unwired: 8 in, 4 out]
  n448 = call "AC Voltage Get BW.vi"() -> ()  [unwired: 8 in, 4 out]
  n449 = call "Strain Get Offset Compensation.vi"() -> ()  [unwired: 8 in, 4 out]
  n450 = call "Measure Strain Direct.vi"() -> ()  [unwired: 8 in, 4 out]
  n451 = call "Scale Get Function.vi"() -> ()  [unwired: 8 in, 4 out]
  n452 = call "Digitizer Scan Fetch FFT Magnitude.vi"() -> ()  [unwired: 12 in, 4 out]
  n453 = call "Scan Get Statistic All.vi"() -> ()  [unwired: 8 in, 4 out]
  n454 = call "Temperature Get Aperture Enabled.vi"() -> ()  [unwired: 8 in, 4 out]
  n455 = call "RTD 4Wire Get Reference Enabled.vi"() -> ()  [unwired: 8 in, 4 out]
  n456 = call "Measure Digital Input.vi"() -> ()  [unwired: 8 in, 4 out]
  n457 = call "DC Current Get Zero Auto.vi"() -> ()  [unwired: 8 in, 4 out]
  n458 = call "Get Minimum Time.vi"() -> ()  [unwired: 8 in, 4 out]
  n459 = call "DC Voltage Get Range Auto.vi"() -> ()  [unwired: 8 in, 4 out]
  n460 = call "Resistance Get Range.vi"() -> ()  [unwired: 8 in, 4 out]
  n461 = call "Single Channel Resistance Get Range.vi"() -> ()  [unwired: 8 in, 4 out]
  n462 = call "Single Channel DC Voltage Get Range.vi"() -> ()  [unwired: 8 in, 4 out]
  n463 = call "AC Voltage Get Range.vi"() -> ()  [unwired: 8 in, 4 out]
  n464 = call "Digitizer Strain Get Voltage Range.vi"() -> ()  [unwired: 8 in, 4 out]
  n465 = call "Strain Get NPLC.vi"() -> ()  [unwired: 8 in, 4 out]
  n466 = call "Measure Strain Direct 4Wire.vi"() -> ()  [unwired: 8 in, 4 out]
  n467 = call "Scale Get dBm Reference.vi"() -> ()  [unwired: 8 in, 4 out]
  n468 = call "Digitizer Scan Fetch Data.vi"() -> ()  [unwired: 12 in, 4 out]
  n469 = call "Measure DC Current.vi"() -> ()  [unwired: 8 in, 4 out]
  n470 = call "Get Peak To Peak.vi"() -> ()  [unwired: 8 in, 4 out]
  n471 = call "DC Voltage Get Zero Auto.vi"() -> ()  [unwired: 8 in, 4 out]
  n472 = call "Resistance Get Range Auto.vi"() -> ()  [unwired: 8 in, 4 out]
  n473 = call "Single Channel Resistance 4Wire Get Range.vi"() -> ()  [unwired: 8 in, 4 out]
  n474 = call "Comparison Get Enabled.vi"() -> ()  [unwired: 8 in, 4 out]
  n475 = call "AC Voltage Get Range Auto.vi"() -> ()  [unwired: 8 in, 4 out]
  n476 = call "Digitizer Strain Get Unstrained Offset.vi"() -> ()  [unwired: 8 in, 4 out]
  n477 = call "Strain Get Gauge Resistance.vi"() -> ()  [unwired: 8 in, 4 out]
  n478 = call "Scale Get dB Reference.vi"() -> ()  [unwired: 8 in, 4 out]
  n479 = call "Digitizer Scan Fetch Statistics.vi"() -> ()  [unwired: 12 in, 4 out]
  n480 = call "Statistics Get Standard Deviation.vi"() -> ()  [unwired: 8 in, 4 out]
  n481 = call "Measure DC Voltage.vi"() -> ()  [unwired: 8 in, 4 out]
  n482 = call "Resistance Get Zero Auto.vi"() -> ()  [unwired: 8 in, 4 out]
  n483 = call "Get Mask.vi"() -> ()  [unwired: 8 in, 4 out]
  n484 = call "Digitizer Strain Get Excitation Voltage.vi"() -> ()  [unwired: 8 in, 4 out]
  n485 = call "Strain Get Gauge Factor.vi"() -> ()  [unwired: 8 in, 4 out]
  n486 = call "Scale Get Auto Reference Enabled.vi"() -> ()  [unwired: 8 in, 4 out]
  n487 = call "Measure Resistance.vi"() -> ()  [unwired: 8 in, 4 out]
  n488 = call "Get Pattern Data.vi"() -> ()  [unwired: 8 in, 4 out]
  n489 = call "Digitizer Strain Get Poisson Ratio.vi"() -> ()  [unwired: 8 in, 4 out]
  n490 = call "Get Alpha.vi"() -> ()  [unwired: 8 in, 4 out]
  n491 = call "Thermocouple Get Check Enabled.vi"() -> ()  [unwired: 8 in, 4 out]
  n492 = call "Thermistor 4Wire Get Reference Enabled.vi"() -> ()  [unwired: 8 in, 4 out]
  n493 = call "Strain Get Excitation Voltage.vi"() -> ()  [unwired: 8 in, 4 out]
  n494 = call "Comparison Get Type.vi"() -> ()  [unwired: 8 in, 4 out]
  n495 = call "Digitizer Strain Get Gauge Factor.vi"() -> ()  [unwired: 8 in, 4 out]
  n496 = call "Thermistor 4Wire Get Probe Type.vi"() -> ()  [unwired: 8 in, 4 out]
  n497 = call "RTD Get Nominal Resistance.vi"() -> ()  [unwired: 8 in, 4 out]
  n498 = call "Get Ref Junction Source.vi"() -> ()  [unwired: 8 in, 4 out]
  n499 = call "Strain Get Excitation Type.vi"() -> ()  [unwired: 8 in, 4 out]
  n500 = call "Thermistor 4Wire Get Low Power.vi"() -> ()  [unwired: 8 in, 4 out]
  n501 = call "RTD Get Offset Compensation.vi"() -> ()  [unwired: 8 in, 4 out]
  n502 = call "Get Ref Junction Temperature.vi"() -> ()  [unwired: 8 in, 4 out]
  n503 = call "Strain Get Aperture.vi"() -> ()  [unwired: 8 in, 4 out]
  n504 = call "Digital Get DAC Output Mode.vi"() -> ()  [unwired: 8 in, 4 out]
  n505 = call "Digitizer Scan Sample Get Rate.vi"() -> ()  [unwired: 8 in, 4 out]
  n506 = call "Measure DAC Sense.vi"() -> ()  [unwired: 8 in, 4 out]
  n507 = call "Resistance 4Wire Get Aperture.vi"() -> ()  [unwired: 8 in, 4 out]
  n508 = call "Resistance 4Wire Get Offset Compensation.vi"() -> ()  [unwired: 8 in, 4 out]
  n509 = call "Measure Thermistor 4Wire.vi"() -> ()  [unwired: 8 in, 4 out]
  n510 = call "Measure RTD.vi"() -> ()  [unwired: 8 in, 4 out]
  n511 = call "Thermocouple Get Type.vi"() -> ()  [unwired: 8 in, 4 out]
  n512 = call "Strain Get Aperture Enabled.vi"() -> ()  [unwired: 8 in, 4 out]
  n513 = call "Digitizer Scan Sample Get Pre Trigger Count.vi"() -> ()  [unwired: 8 in, 4 out]
  n514 = call "Digital Get DAC Output Lock.vi"() -> ()  [unwired: 8 in, 4 out]
  n515 = call "Measure DAC Output.vi"() -> ()  [unwired: 8 in, 4 out]
  n516 = call "Resistance 4Wire Get Aperture Enabled.vi"() -> ()  [unwired: 8 in, 4 out]
  n517 = call "Resistance 4Wire Get Range.vi"() -> ()  [unwired: 8 in, 4 out]
  n518 = call "RTD Get Reference Enabled.vi"() -> ()  [unwired: 8 in, 4 out]
  n519 = call "Measure Strain Quarter Bridge.vi"() -> ()  [unwired: 8 in, 4 out]
  n520 = call "Read Ref Junction Temperature.vi"() -> ()  [unwired: 8 in, 4 out]
  n521 = call "Digitizer Scan Sample Get Count.vi"() -> ()  [unwired: 8 in, 4 out]
  n522 = call "Digital Get DAC Current.vi"() -> ()  [unwired: 8 in, 4 out]
  n523 = call "Resistance 4Wire Get Low Power.vi"() -> ()  [unwired: 8 in, 4 out]
  n524 = call "Resistance 4Wire Get Range Auto.vi"() -> ()  [unwired: 8 in, 4 out]
  n525 = call "Measure Thermocouple.vi"() -> ()  [unwired: 8 in, 4 out]
  n526 = call "Digital Get DAC Voltage.vi"() -> ()  [unwired: 8 in, 4 out]
  n527 = call "Resistance 4Wire Get NPLC.vi"() -> ()  [unwired: 8 in, 4 out]
  n528 = call "Measure Resistance 4Wire.vi"() -> ()  [unwired: 8 in, 4 out]
  n529 = call "Calibrate.vi"() -> ()  [unwired: 9 in, 3 out]
  n530 = call "Disable.vi"() -> ()  [unwired: 10 in, 2 out]
  n531 = call "Set Daily Interval Time.vi"() -> ()  [unwired: 10 in, 2 out]
  n532 = call "Secure Instrument.vi"() -> ()  [unwired: 10 in, 2 out]
  n533 = call "System Get Temperature.vi"() -> ()  [unwired: 9 in, 3 out]
  n534 = call "Error Message.vi"() -> ()  [unwired: 9 in, 3 out]
  n535 = call "Get Module State.vi"() -> ()  [unwired: 9 in, 3 out]
  n536 = call "Unsecure Instrument.vi"() -> ()  [unwired: 10 in, 2 out]
  n537 = call "Error-Query.vi"() -> ()  [unwired: 8 in, 4 out]
  n538 = call "System Auto Calibration Date Time.vi"() -> ()  [unwired: 9 in, 3 out]
  n539 = call "Calibration Temperature.vi"() -> ()  [unwired: 9 in, 3 out]
  n540 = call "Reset.vi"() -> ()  [unwired: 10 in, 2 out]
  n541 = call "Calibration Store.vi"() -> ()  [unwired: 10 in, 2 out]
  n542 = call "Reset With Defaults.vi"() -> ()  [unwired: 10 in, 2 out]
  n543 = call "Calibration ADC Circuit.vi"() -> ()  [unwired: 9 in, 3 out]
  n544 = call "Revision Query.vi"() -> ()  [unwired: 8 in, 4 out]
  n545 = call "Self-Test.vi"() -> ()  [unwired: 8 in, 4 out]
  n546 = call "Close.vi"() -> ()  [unwired: 11 in, 1 out]
